vi "List.vi"(8 "error in (no error)":errorcluster) -> (0 "error out":errorcluster, 1 "Ports #":i32, 2 "Serial Ports":string[](array[string]), 5 "Success?":bool)   [LabVIEW 2013, in "Thorlabs_MC2000B.lvlib"]
uses:
  <instrlib>/Thorlabs_MC2000B/Thorlabs_MC2000B.lvlib
  <instrlib>/Thorlabs_MC2000B/Library/MC2000CommandLibWin64.dll
  <instrlib>/Thorlabs_MC2000B/Library/MC2000CommandLibWin32.dll
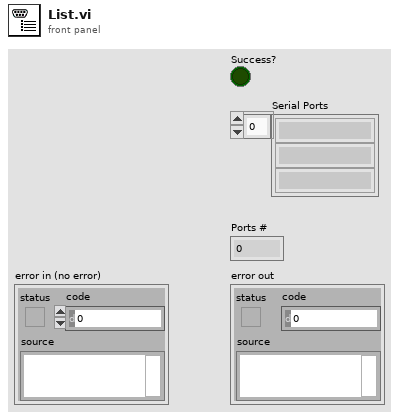
[diagram p1: front panel]
types:
  T1 = cluster{"offset past number":i32, "Name":string}[]
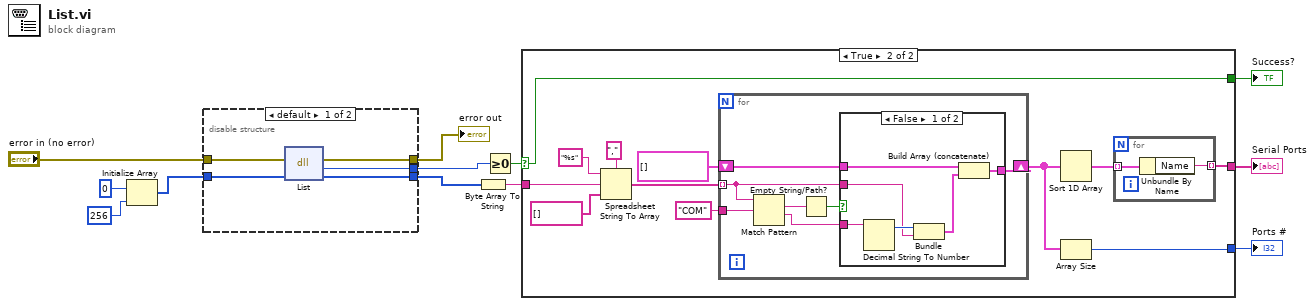
[diagram p0: block diagram]
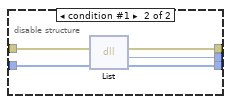
[diagram p2: hidden frame]
diagram:
  n1 = Initialize Array(u8 0 ("element"), 256 ("Var")) -> (w4:u8[])
  n2 = disable-structure shown="default" {
    disable-tunnel: [w17 w22] -> w10
    disable-tunnel: "error in (no error)" -> [w16 w21]
    disable-tunnel: [w15 w20] -> w6
    disable-tunnel: w4 -> [w14 w19]
    disable-tunnel: [w13 w18] -> w2
    frame condition #0 (active) {
      n3 = dll-call lib="C:/Program Files (x86)/National Instruments/LabVIEW 2013/instr.lib/Thorlabs_MC2000B/Library/MC2000CommandLibWin32.dll" fn="List"(error in=w16, "nPort"=w14) -> (error out=w15:errorcluster, "return type"=w17:i32, "nPort"=w13:u8[])  [unwired: 2 in, 1 out]
    }
    frame condition #1 {
      n4 = dll-call lib="D:/Program Files/National Instruments/LabVIEW 2011/instr.lib/Thorlabs_MC2000B/Library/MC2000CommandLibWin64.dll" fn="List"(error in=w21, "nPort"=w19) -> (error out=w20:errorcluster, "return type"=w22:i32, "nPort"=w18:u8[])  [unwired: 2 in, 1 out]
    }
  }
  "error out" <- w6
  n5 = Byte Array To String(unsigned byte array=w2) -> (string=w1:string)
  n6 = Greater Or Equal To 0?(x=w10) -> (x >= 0?=w9:bool)
  n7 = case shown="True" w9 {
    selector: w9 -> [w23 w29]
    tunnel: [_ w24] -> w12
    tunnel: [_ w30] -> w11
    tunnel: [w23 w29] -> w8
    tunnel: w1 -> [_ w28]
    frame False {
    }
    frame True {
      n8 = Spreadsheet String To Array(delimiter (Tab)=",", format string="%s", spreadsheet string=w28, array type (2D Dbl)=string[] []) -> (array=w32:string[])
      n9 = for {
        tunnel: w32 -> [w41] mode=indexing
        shift-right: [w44] -> w31
        shift-left: cluster{"ID":i32, "Name":string}[] [] -> [w43]
        tunnel: "COM" ("regular expression") -> [w40]
        n10 = Match Pattern(string=w41, regular expression=w40) -> (match substring=w39:string, after substring=w38:string)  [unwired: 1 in, 2 out]
        n11 = Empty String/Path?(string/path=w39) -> (empty?=w42:bool)
        n12 = case shown="False" w42 {
          tunnel: w41 -> [w46 _]
          tunnel: [w50 w51] -> w44
          tunnel: w43 -> [w49 w51]
          tunnel: w38 -> [w48 _]
          frame False {
            n13 = Decimal String To Number(string=w48) -> (offset past number=w47:i32)  [unwired: 2 in, 1 out]
            n14 = Bundle("offset past number"=w47, w46) -> (w45:cluster{"offset past number":i32, string})  [unwired: 1 in]
            n15 = Build Array (concatenate)(w49, w45) -> (w50:T1)
          }
          frame True {
          }
        }
      }
      n16 = Sort 1D Array(array=w31) -> (sorted array=w25:cluster{"ID":i32, "Name":string}[])
      n17 = Array Size(array=w31) -> (size(s)=w30:i32)
      n18 = for {
        tunnel: w25 -> [w37] mode=indexing
        tunnel: [w36] -> w24 mode=indexing
        n19 = Unbundle By Name(w37) -> ("Name"=w36:string)
      }
    }
  }
  "Serial Ports" <- w12
  "Ports #" <- w11
  "Success?" <- w8
